vi "laser_diode.vi"() -> ()   [LabVIEW 2018]
uses:
  enum_states.ctl
panel:
  out "Temperature Control LED":bool
  out "Temperature Control":string
  out "Laser Diode Temperature Lower Limit [°C]":dbl
  out "Laser Diode Current Lower Limit [mA]":dbl
  out "Laser Diode Temperature Upper Limit [°C]":dbl caption="Laser Diode Current Limit"
  in  "Set temperature":bool
  out "Output On?":bool
  in  "On/Off":bool
  out "Initialized?":bool
  in  "Close all":bool
  in  "Set current":bool
  out "Laser Diode Current Upper Limit [mA]":dbl caption="Laser Diode Current Limit"
  in  "Start initialization":bool
  in  "Stusa tutto My1":bool
  # "EMERGENCY BUTTON"
  # "INITIALIZE THE SYSTEM: ONLY WHEN LIGHT IS GREEN YOU CAN GO ON"
  # "CONTROL THE SYSTEM"
  # "SWITCH ON/OFF LASER"
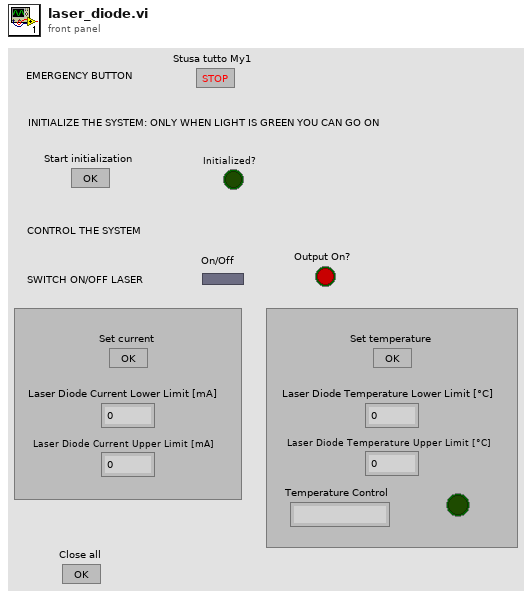
[diagram p1: front panel]
types:
  T1 = typedef "enum_states.ctl" = enum16{"initialize", "wait", "set current", "waiting current", "set temperature", "waiting temperature", "close"}
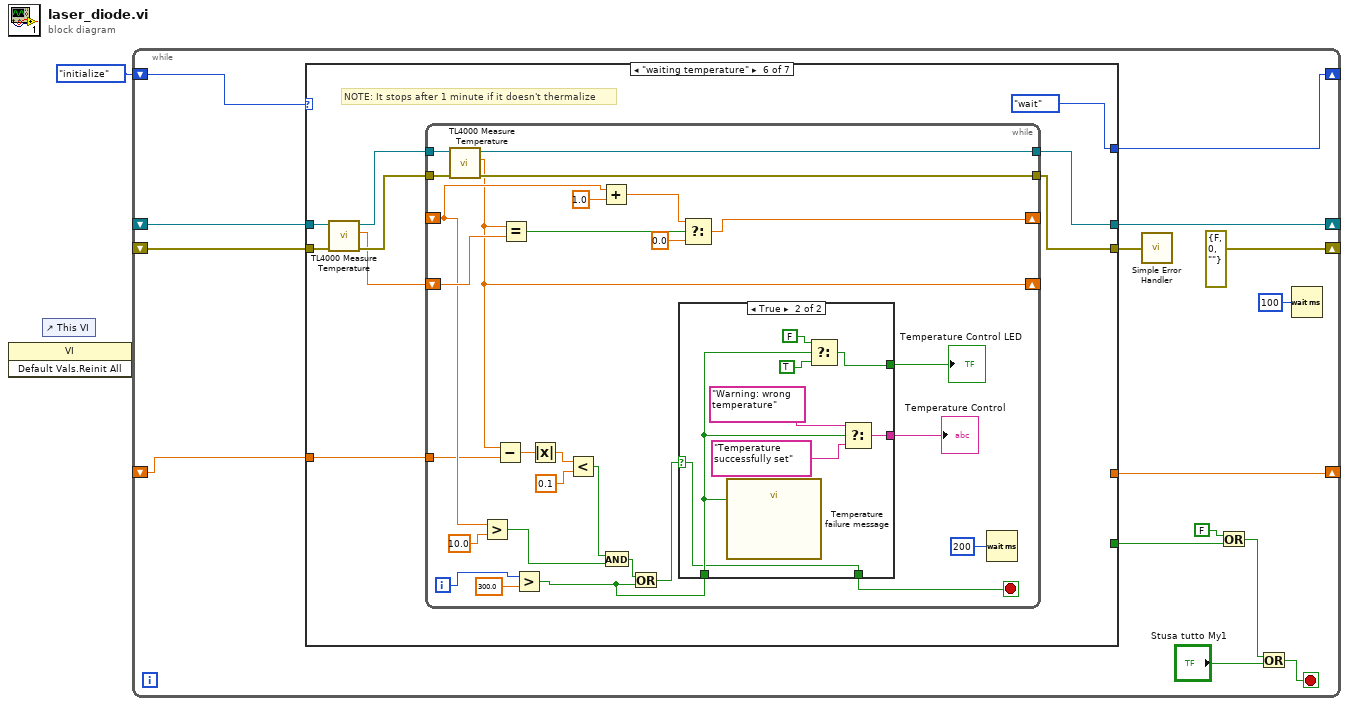
[diagram p0: block diagram]
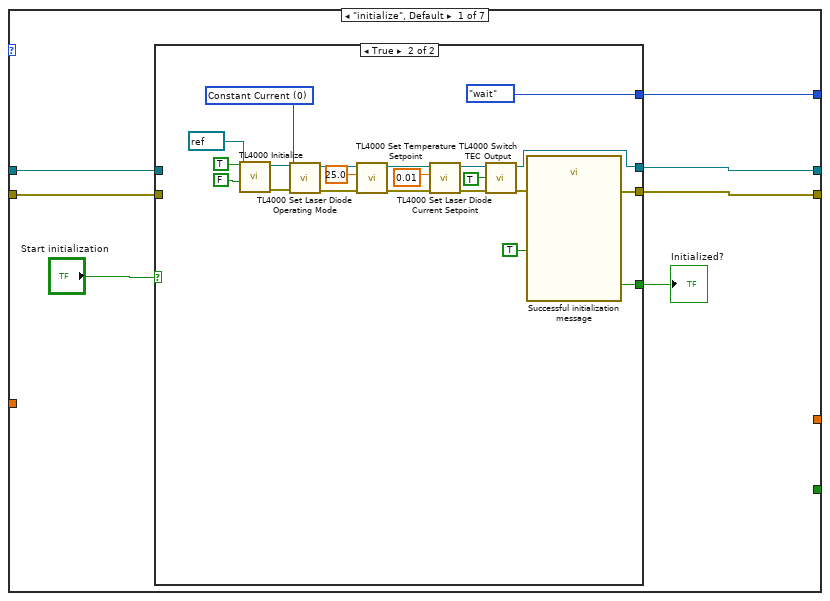
[diagram p2: hidden frame]
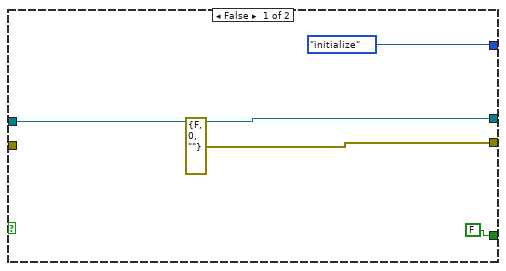
[diagram p3: hidden frame]
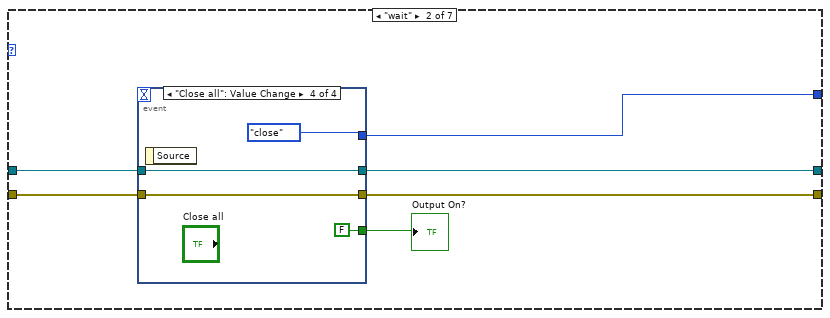
[diagram p4: hidden frame]
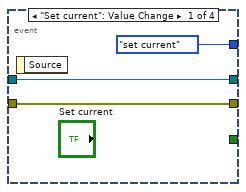
[diagram p5: hidden frame]
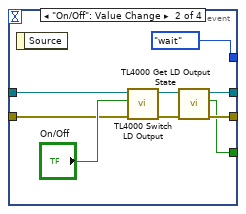
[diagram p6: hidden frame]
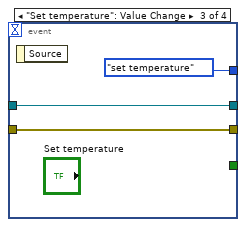
[diagram p7: hidden frame]
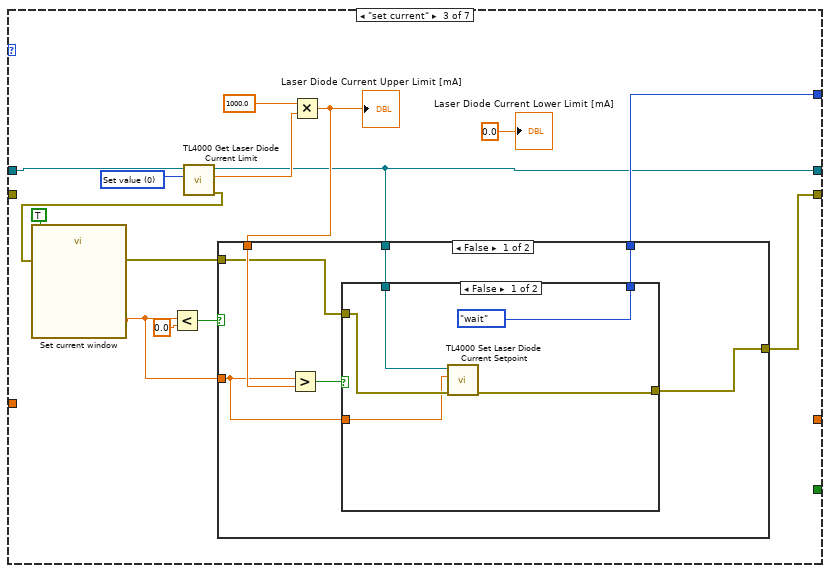
[diagram p8: hidden frame]
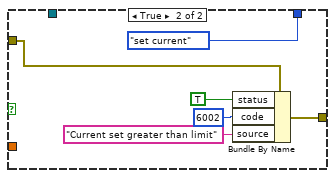
[diagram p9: hidden frame]
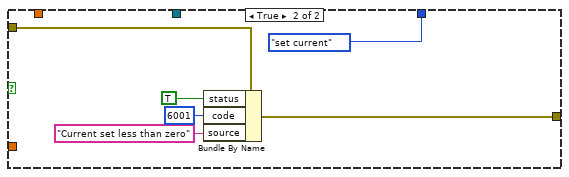
[diagram p10: hidden frame]
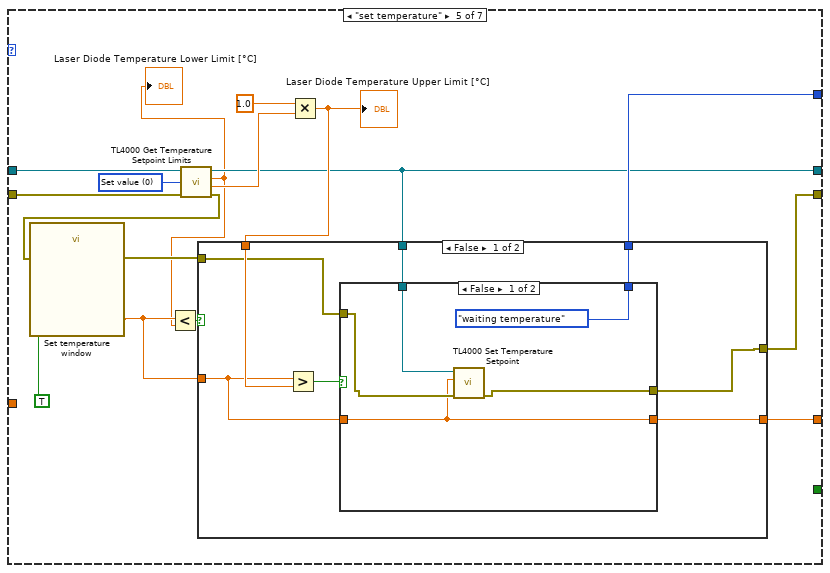
[diagram p12: hidden frame]
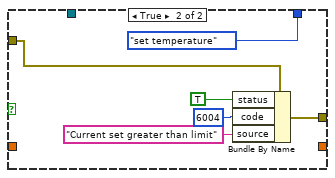
[diagram p13: hidden frame]
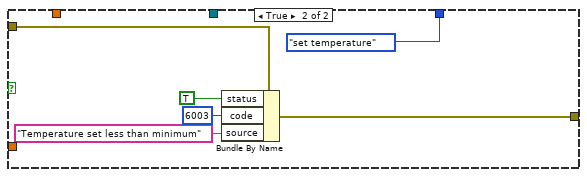
[diagram p14: hidden frame]
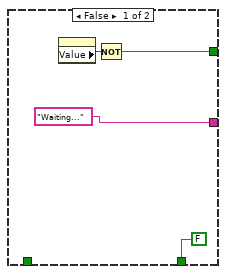
[diagram p15: hidden frame]
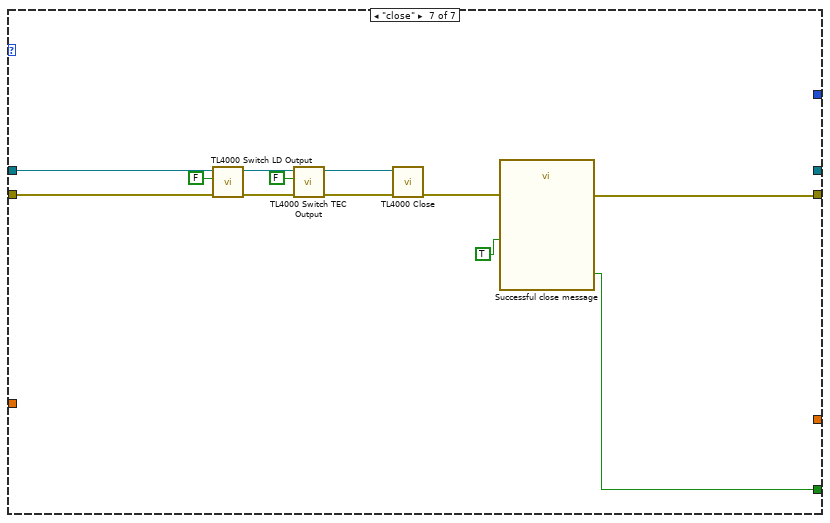
[diagram p16: hidden frame]
diagram:
  n1 = invoke class="VI" method="Default Vals.Reinit All"() -> ()  [unwired: 3 in, 3 out]
  n2 = control-ref of="This VI"() -> ()  [unwired: 1 out]
  n3 = while {
    shift-right: [w7] -> _
    shift-left: enum_states."initialize" -> [w8]
    shift-right: [errorcluster {"status"=FALSE, "code"=0, "source"=""} ("error constant")] -> _
    shift-left: _ -> [w5]
    shift-right: [w13] -> _
    shift-left: _ -> [w6]
    shift-right: [w3] -> _
    shift-left: _ -> [w2]
    stop <- w16 stop-if-true
    n4 = case shown="\"waiting temperature\"" w8 {
      tunnel: [w20 w54 w81 _ w123 enum_states."wait" _] -> w7
      tunnel: [w21 w51 w75 w114 w117 w164 _] -> w13
      tunnel: [w22 w50 w83 w113 w124 w163 w207] -> w12
      tunnel: w6 -> [w19 w53 w88 w114 w122 w162 w216]
      tunnel: w5 -> [w18 w52 _ w113 w121 w161 w215]
      tunnel: [_ _ _ _ _ _ w205] -> w4
      tunnel: [_ _ _ _ w115 _ _] -> w3
      tunnel: w2 -> [_ _ _ _ _ w157 _]
      frame "initialize", Default {
        n5 = case shown="True" "Start initialization" {
          tunnel: [w27 w30] -> w21
          tunnel: [errorcluster {"status"=FALSE, "code"=0, "source"=""} ("error constant") w31] -> w22
          tunnel: [enum_states."initialize" enum_states."wait"] -> w20
          tunnel: w19 -> [w27 _]
          tunnel: w18 -> [_ _]
          tunnel: [FALSE ("Initialized?") w28] -> w17
          frame False {
          }
          frame True {
            w43 = i16 0 items=["Constant Current", "Constant Power"] ("Laser Diode Operating Mode (Constant Current)")
            n6 = call <instrlib>:"TL4000 Initialize.vi"("Reset Device (Reset Device)"=FALSE, "ID Query (Do Query)"=TRUE, "resource name"=refnum<visa-resource-name> "USB0::0x1313::0x804F::M00307175::INSTR") -> ("error out"=w44:errorcluster, "instrument handle out"=w45:refnum<visa-resource-name>)  [unwired: 7 in]
            n7 = call <instrlib>:"TL4000 Set Laser Diode Operating Mode.vi"("error in (no error)"=w44, "Laser Diode Operating Mode (Constant Current)"=w43, "instrument handle"=w45) -> ("error out"=w39:errorcluster, "instrument handle out"=w40:refnum<visa-resource-name>)  [unwired: 7 in]
            n8 = call <instrlib>:"TL4000 Set Temperature Setpoint.vi"("error in (no error)"=w39, "Temperature Setpoint (25.0)"=25.0, "instrument handle"=w40) -> ("error out"=w37:errorcluster, "instrument handle out"=w36:refnum<visa-resource-name>)  [unwired: 7 in]
            n9 = call <instrlib>:"TL4000 Set Laser Diode Current Setpoint.vi"("error in (no error)"=w37, "Laser Diode Current Setpoint (0.0)"=0.01, "instrument handle"=w36) -> ("error out"=w33:errorcluster, "instrument handle out"=w34:refnum<visa-resource-name>)  [unwired: 7 in]
            n10 = call <instrlib>:"TL4000 Switch TEC Output.vi"("error in (no error)"=w33, "TEC Output (Off)"=TRUE, "instrument handle"=w34) -> ("error out"=w32:errorcluster, "instrument handle out"=w30:refnum<visa-resource-name>)  [unwired: 7 in]
            n11 = call "Successful initialization message"("error in (no error)"=w32, "Enable"=TRUE) -> ("error out"=w31:errorcluster, "OK"=w28:bool)  [unwired: 8 in]
          }
        }
        "Initialized?" <- w17
      }
      frame "wait" {
        n12 = event shown="[3] \"Close all\": Value Change" {
          selector: _ -> [_ _ _ _]
          dyn-events: _ -> [_ _ _ _]
          timeout: _ -> [_ _ _ _]
          tunnel: [enum_states."set current" enum_states."wait" enum_states."set temperature" enum_states."close"] -> w54
          tunnel: [_ w58 _ FALSE ("On/Off")] -> w49
          tunnel: w53 -> [w56 w64 w68 w72]
          tunnel: [w56 w60 w68 w72] -> w51
          tunnel: w52 -> [w55 w63 w69 w71]
          tunnel: [w55 w59 w69 w71] -> w50
          event "Set current": Value Change {
            n13 = event-data() -> ()  [unwired: 1 in, 1 out]
          }
          event "On/Off": Value Change {
            n14 = event-data() -> ()  [unwired: 1 in, 1 out]
            n15 = call <instrlib>:"TL4000 Switch LD Output.vi"("error in (no error)"=w63, "LD Output (Off)"="On/Off", "instrument handle"=w64) -> ("error out"=w62:errorcluster, "instrument handle out"=w61:refnum<visa-resource-name>)  [unwired: 7 in]
            n16 = call <instrlib>:"TL4000 Get LD Output State.vi"("error in (no error)"=w62, "instrument handle"=w61) -> ("error out"=w59:errorcluster, "LD Output"=w58:bool, "instrument handle out"=w60:refnum<visa-resource-name>)  [unwired: 7 in]
          }
          event "Set temperature": Value Change {
            n17 = event-data() -> ()  [unwired: 1 in, 1 out]
          }
          event "Close all": Value Change {
            n18 = event-data() -> ()  [unwired: 1 in, 1 out]
          }
        }
        "Output On?" <- w49
      }
      frame "set current" {
        w87 = i16 0 items=["Set value", "Minimum value", "Maximum value"] ("Attribute (Set value)")
        n19 = call <instrlib>:"TL4000 Get Laser Diode Current Limit.vi"("Attribute (Set value)"=w87, "instrument handle"=w88) -> ("error out"=w79:errorcluster, "Laser Diode Current Limit"=w82:dbl, "instrument handle out"=w75:refnum<visa-resource-name>)  [unwired: 7 in]
        n20 = call "Set current window"("Enable"=TRUE, "error in (no error)"=w79) -> ("Set current:"=w77:dbl, "error out"=w78:errorcluster)  [unwired: 15 in, 1 out]
        n21 = Less?(x=w77, y=0.0) -> (x < y?=w84:bool)
        n22 = Multiply(x=1000.0, y=w82) -> (x*y=w76:dbl)
        "Laser Diode Current Upper Limit [mA]" <- w76
        n23 = case shown="False" w84 {
          tunnel: [w93 w109] -> w83
          tunnel: w77 -> [w90 _]
          tunnel: w76 -> [w95 _]
          tunnel: [w92 enum_states."set current"] -> w81
          tunnel: w78 -> [w91 w108]
          tunnel: w75 -> [w89 _]
          frame False {
            n24 = Greater?(x=w90, y=w95) -> (0:w94:bool)
            n25 = case shown="False" w94 {
              tunnel: [w98 w103] -> w93
              tunnel: [enum_states."wait" enum_states."set current"] -> w92
              tunnel: w91 -> [w99 w102]
              tunnel: w90 -> [w96 _]
              tunnel: w89 -> [w97 _]
              frame False {
                n26 = call <instrlib>:"TL4000 Set Laser Diode Current Setpoint.vi"("error in (no error)"=w99, "Laser Diode Current Setpoint (0.0)"=w96, "instrument handle"=w97) -> ("error out"=w98:errorcluster)  [unwired: 7 in, 1 out]
              }
              frame True {
                n27 = Bundle By Name(cluster=w102, "status"=TRUE, "code"=6002, "source"="Current set greater than limit") -> (w103:errorcluster)
              }
            }
          }
          frame True {
            n28 = Bundle By Name(cluster=w108, "status"=TRUE, "code"=6001, "source"="Current set less than zero") -> (w109:errorcluster)
          }
        }
        "Laser Diode Current Lower Limit [mA]" <- 0.0 ("Laser Diode Current Lower Limit [mA]")
      }
      frame "waiting current" {
      }
      frame "set temperature" {
        w120 = i16 0 items=["Set value", "Minimum value", "Maximum value"] ("Attribute (Set value)")
        n29 = call <instrlib>:"TL4000 Get Temperature Setpoint Limits.vi"("error in (no error)"=w121, "Attribute (Set value)"=w120, "instrument handle"=w122) -> ("error out"=w119:errorcluster, "Setpoint High Limit"=w118:dbl, "Setpoint Low Limit"=w116:dbl, "instrument handle out"=w117:refnum<visa-resource-name>)  [unwired: 5 in]
        "Laser Diode Temperature Lower Limit [°C]" <- w116
        n30 = call "Set temperature window"("Enable"=TRUE, "error in (no error)"=w119) -> ("Set temperature:"=w126:dbl, "error out"=w127:errorcluster)  [unwired: 15 in, 1 out]
        n31 = Less?(x=w126, y=w116) -> (x < y?=w129:bool)
        n32 = Multiply(x=1.0, y=w118) -> (x*y=w125:dbl)
        "Laser Diode Temperature Upper Limit [°C]" <- w125
        n33 = case shown="False" w129 {
          tunnel: [w136 w152] -> w124
          tunnel: w126 -> [w133 _]
          tunnel: w125 -> [w138 _]
          tunnel: w127 -> [w134 w151]
          tunnel: [w135 enum_states."set temperature"] -> w123
          tunnel: w117 -> [w132 _]
          tunnel: [w131 _] -> w115
          frame False {
            n34 = Greater?(x=w133, y=w138) -> (0:w137:bool)
            n35 = case shown="False" w137 {
              tunnel: [w141 w146] -> w136
              tunnel: [enum_states."waiting temperature" enum_states."set temperature"] -> w135
              tunnel: w134 -> [w142 w145]
              tunnel: w133 -> [w139 _]
              tunnel: w132 -> [w140 _]
              tunnel: [w139 _] -> w131
              frame False {
                n36 = call <instrlib>:"TL4000 Set Temperature Setpoint.vi"("error in (no error)"=w142, "Temperature Setpoint (25.0)"=w139, "instrument handle"=w140) -> ("error out"=w141:errorcluster)  [unwired: 7 in, 1 out]
              }
              frame True {
                n37 = Bundle By Name(cluster=w145, "status"=TRUE, "code"=6004, "source"="Current set greater than limit") -> (w146:errorcluster)
              }
            }
          }
          frame True {
            n38 = Bundle By Name(cluster=w151, "status"=TRUE, "code"=6003, "source"="Temperature set less than minimum") -> (w152:errorcluster)
          }
        }
      }
      frame "waiting temperature" {
        # "NOTE: It stops after 1 minute if it doesn't thermalize"
        n39 = call <instrlib>:"TL4000 Measure Temperature.vi"("error in (no error)"=w161, "instrument handle"=w162) -> ("error out"=w160:errorcluster, "Temperature"=w159:dbl, "instrument handle out"=w158:refnum<visa-resource-name>)  [unwired: 7 in]
        n40 = while {
          tunnel: w160 -> [w192]
          tunnel: [w191] -> w164
          tunnel: [w190] -> w163
          shift-right: [w188] -> _
          shift-left: _ -> [w179]
          shift-right: [w177] -> _
          shift-left: w159 -> [w183]
          tunnel: w158 -> [w178]
          tunnel: w157 -> [w176]
          i -> [w181]
          stop <- w168 stop-if-true
          n41 = call <instrlib>:"TL4000 Measure Temperature.vi"("error in (no error)"=w192, "instrument handle"=w178) -> ("error out"=w190:errorcluster, "Temperature"=w177:dbl, "instrument handle out"=w191:refnum<visa-resource-name>)  [unwired: 7 in]
          n42 = Greater?(x=w179, y=10.0) -> (0:w171:bool)
          n43 = Subtract(x=w177, y=w176) -> (x-y=w175:dbl)
          n44 = Equal?(x=w177, y=w183) -> (x = y?=w186:bool)
          n45 = Greater?(x=w181, y=300.0) -> (0:w165:bool)
          n46 = Absolute Value(x=w175) -> (abs(x)=w174:dbl)
          n47 = Less?(x=w174, y=0.1) -> (x < y?=w172:bool)
          n48 = Add(x=w179, y=1.0) -> (x+y=w184:dbl)
          n49 = And(x=w172, y=w171) -> (x .and. y?=w170:bool)
          n50 = Or(x=w170, y=w165) -> (x .or. y?=w169:bool)
          n51 = case shown="True" w169 {
            selector: w169 -> [_ w197]
            tunnel: [FALSE w197] -> w168
            tunnel: [w194 w204] -> w167
            tunnel: ["Waiting..." ("Temperature Control") w203] -> w166
            tunnel: w165 -> [_ w202]
            frame False {
              n52 = property on="Temperature Control LED" class="Bool (strict)"() -> ("Value"=w196:bool)  [unwired: 2 in, 2 out]
              n53 = Not(x=w196) -> (.not. x?=w194:bool)
            }
            frame True {
              n54 = call "Temperature failure message"("Enable"=w202) -> ()  [unwired: 9 in, 2 out]
              n55 = Select(t=FALSE, s=w202, f=TRUE) -> (s? t:f=w204:bool)
              n56 = Select(t="Warning: wrong temperature", s=w202, f="Temperature successfully set") -> (s? t:f=w203:string)
            }
          }
          "Temperature Control LED" <- w167
          "Temperature Control" <- w166
          n57 = Select(t=w184, s=w186, f=0.0) -> (s? t:f=w188:dbl)
          n58 = Wait (ms)(milliseconds to wait=u32 200) -> ()  [unwired: 1 out]
        }
      }
      frame "close" {
        n59 = call <instrlib>:"TL4000 Switch LD Output.vi"("error in (no error)"=w215, "LD Output (Off)"=FALSE, "instrument handle"=w216) -> ("error out"=w212:errorcluster, "instrument handle out"=w213:refnum<visa-resource-name>)  [unwired: 7 in]
        n60 = call <instrlib>:"TL4000 Switch TEC Output.vi"("error in (no error)"=w212, "TEC Output (Off)"=FALSE, "instrument handle"=w213) -> ("error out"=w209:errorcluster, "instrument handle out"=w210:refnum<visa-resource-name>)  [unwired: 7 in]
        n61 = call <instrlib>:"TL4000 Close.vi"("error in (no error)"=w209, "instrument handle"=w210) -> ("error out"=w208:errorcluster)  [unwired: 9 in]
        n62 = call "Successful close message"("error in (no error)"=w208, "Enable"=TRUE) -> ("error out"=w207:errorcluster, "OK"=w205:bool)  [unwired: 8 in]
      }
    }
    n63 = call <vilib>:"Simple Error Handler.vi"("error in (no error)"=w12) -> ()  [unwired: 4 in, 5 out]
    n64 = Or(x=FALSE, y=w4) -> (x .or. y?=w11:bool)
    n65 = Or(x=w11, y="Stusa tutto My1") -> (x .or. y?=w16:bool)
    n66 = Wait (ms)(milliseconds to wait=u32 100) -> ()  [unwired: 1 out]
  }
